vi "visible.vi"(0 "visible":bool, 1 "Array":refnum<vi>[](array[refnum])) -> ()   [LabVIEW 2013]
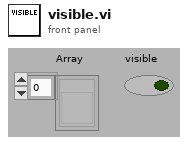
[diagram p1: front panel]
types:
  T1 = enum8{"Enabled", "Disabled", "Disabled and Grayed Out"}
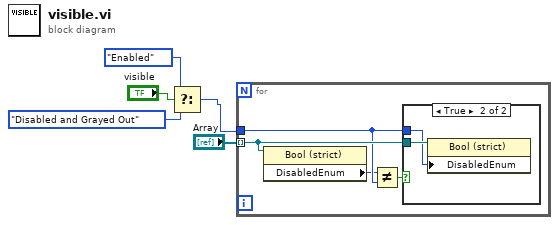
[diagram p0: block diagram]
diagram:
  n1 = Select(t=T1."Enabled" ("Disabled"), s="visible", f=T1."Disabled and Grayed Out" ("Disabled")) -> (s? t:f=w1:T1)
  n2 = for {
    tunnel: "Array" -> [w9] mode=indexing
    tunnel: w1 -> [w8]
    n3 = property class="Bool (strict)"(reference=w9) -> ("DisabledEnum"=w7:T1)  [unwired: 1 in, 2 out]
    n4 = Not Equal?(x=w7, y=w8) -> (x != y?=w6:bool)
    n5 = case shown="True" w6 {
      tunnel: w9 -> [_ w11]
      tunnel: w8 -> [_ w10]
      frame False {
      }
      frame True {
        n6 = property class="Bool (strict)"(reference=w11, "DisabledEnum"=w10) -> ()  [unwired: 1 in, 2 out]
      }
    }
  }
